vi "stop vis.vi"() -> (0 "Abort error":errorcluster)   [LabVIEW 2016, in "main.lvlib"]
doc: "This vi stops each vi for the main control vi subpanel"
uses:
  main.lvlib
  Beam Line Sections/R45.vi
  Beam Line Sections/LowEnd.vi
  Beam Line Sections/Source A.vi
  Tools/bpm.vi
  Tools/scan injector.vi
  Tools/flat top.vi
  Tools/terminal voltage readbacks.vi
  Tools/injector magnet.vi
  Tools/Scale.vi
  Tools/small current measurement.vi
  Tools/GFM monitor.vi
  Tools/Scale - molecular.vi
  High energy end/High energy llb.lvlib
  controls/beamline sections.lvlib
  R30/R30  library.lvlib
  Transmission/transmission.lvlib
  low energy end/Low energy end/Low energy end llb.lvlib
  Features/features/features.lvlib
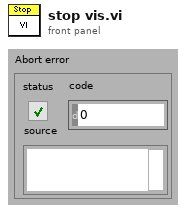
[diagram p1: front panel]
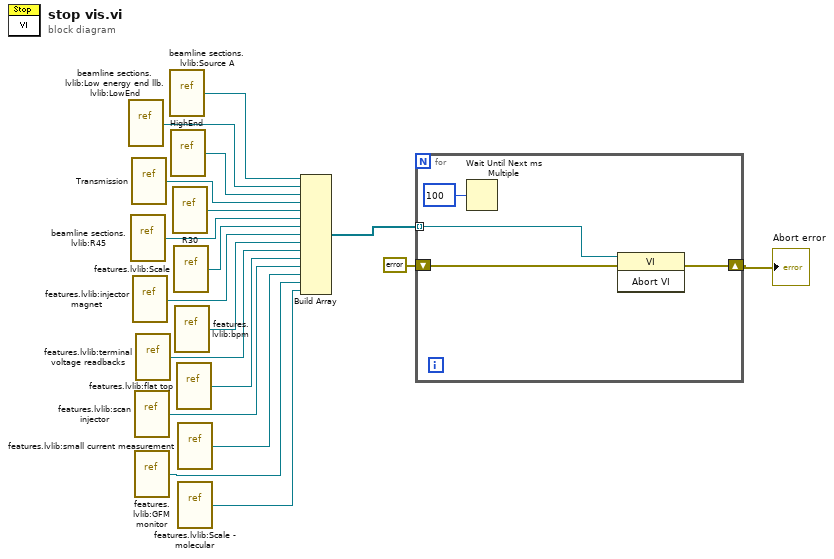
[diagram p0: block diagram]
diagram:
  n1 = vi-ref "beamline sections.lvlib:Low energy end llb.lvlib:LowEnd.vi"() -> (w14:refnum<vi>)
  n2 = vi-ref "beamline sections.lvlib:R45.vi"() -> (w18:refnum<vi>)
  n3 = vi-ref "Transmission.vi"() -> (w16:refnum<vi>)
  n4 = vi-ref "features.lvlib:injector magnet.vi"() -> (w9:refnum<vi>)
  n5 = vi-ref "features.lvlib:scan injector.vi"() -> (w5:refnum<vi>)
  n6 = vi-ref "features.lvlib:GFM monitor.vi"() -> (w2:refnum<vi>)
  n7 = vi-ref "features.lvlib:terminal voltage readbacks.vi"() -> (w7:refnum<vi>)
  n8 = vi-ref "beamline sections.lvlib:Source A.vi"() -> (w13:refnum<vi>)
  n9 = vi-ref "HighEnd.vi"() -> (w15:refnum<vi>)
  n10 = vi-ref "R30.vi"() -> (w17:refnum<vi>)
  n11 = vi-ref "features.lvlib:Scale.vi"() -> (w10:refnum<vi>)
  n12 = vi-ref "features.lvlib:bpm.vi"() -> (w8:refnum<vi>)
  n13 = vi-ref "features.lvlib:flat top.vi"() -> (w6:refnum<vi>)
  n14 = vi-ref "features.lvlib:small current measurement.vi"() -> (w4:refnum<vi>)
  n15 = vi-ref "features.lvlib:Scale - molecular.vi"() -> (w1:refnum<vi>)
  n16 = Build Array(w13, w14, w15, w16, w17, w18, w10, w9, w8, w7, w6, w5, w4, w2, w1) -> (w12:refnum<vi>[])
  n17 = for {
    shift-right: [w21] -> w11
    shift-left: errorcluster {"status"=FALSE, "code"=0, "source"=""} ("error out") -> [w20]
    tunnel: w12 -> [w19] mode=indexing
    n18 = Wait Until Next ms Multiple(millisecond multiple=u32 100) -> ()  [unwired: 1 out]
    n19 = invoke class="VI" method="Abort VI"(reference=w19, error in=w20) -> (error out=w21:errorcluster)  [unwired: 1 in, 2 out]
  }
  "Abort error" <- w11
